vi "Create Writer Endpoint.vi"(6 "writer name":string="//localhost/S4ACS_C1_WRITER", 8 "error in (no error)":errorcluster, 9 "reader name":string="S4GUI_C1_READER", 10 "IP":string="//200.131.64.48", 11 "Stream in":refnum<class "Stream.lvclass">) -> (0 "error out":errorcluster, 3 "Stream out":refnum<class "Stream.lvclass">)   [LabVIEW 2018, in "Stream.lvclass"]
uses:
  Stream.lvclass
  Stream.lvclass/Stream.ctl
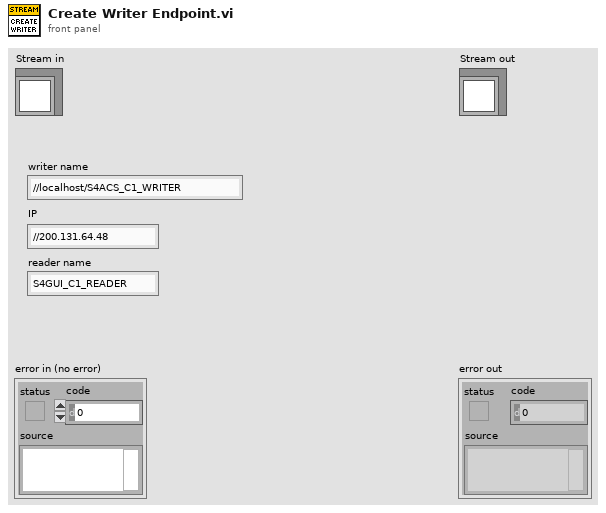
[diagram p1: front panel]
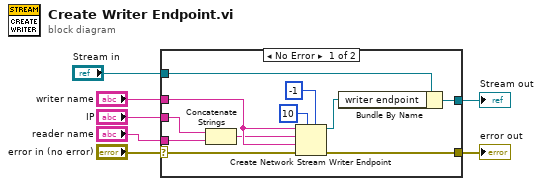
[diagram p0: block diagram]
diagram:
  n1 = case shown="No Error" "error in (no error)" {
    selector: "error in (no error)" -> [w17 w20]
    tunnel: [w18 w20] -> w6
    tunnel: [w14 w19] -> w4
    tunnel: "Stream in" -> [w15 w19]
    tunnel: "IP" -> [w12 _]
    tunnel: "reader name" -> [w9 _]
    tunnel: "writer name" -> [w10 _]
    frame No Error {
      n2 = Concatenate Strings(w12, w9) -> (w8:string)
      n3 = Create Network Stream Writer Endpoint(5:-1 ("timeout in ms (-1)"), 7:10 ("writer buffer size"), 8:w17, 9:w10, 10:w8, 11:w10) -> (0:w18:errorcluster, 3:w11:refnum<k21>)  [unwired: 1 in]
      n4 = Bundle By Name(cluster=w15, "writer endpoint"=w11) -> (w14:refnum<class "Stream.lvclass">)
    }
    frame Error {
    }
  }
  "error out" <- w6
  "Stream out" <- w4
